vi "Autonomous.vi"   [LabVIEW 2018]
doc: "This VI starts when autonomous period begins, and will automatically be terminated when it ends. You can carry out timed or sensor driven operations directly to I/O or to subsystems without needing to return to the caller."
uses:
  <vilib>/Rock Robotics/WPI/Solenoid/WPI_SolenoidValue.ctl
  <vilib>/Rock Robotics/WPI/Utilities/WPI_GetSetVariantRefNum.vi
  <vilib>/Rock Robotics/Network Tables/NT Read String.vi
  Framework/Robot Global Data.vi
types:
  T1 = typedef "WPI_JoystickDevRef.ctl" = cluster{"Device":T2}
  T2 = typedef "WPI_JoystickDeviceEnum.ctl" = enum16{"USB 0", "USB 1", "USB 2", "USB 3", "USB 4", "USB 5"}
  T3 = typedef "WPI_SolenoidValue.ctl" = enum16{"Off", "On", "Forward", "Reverse"}
  T4 = typedef "Command Status Info.ctl" = cluster{"Name":string, "Status":T5, "notifier out":T6}
  T5 = typedef "Completion Status.ctl" = enum16{"Successful", "Aborted", "Incomplete"}
  T6 = typedef "Completion Notifier.ctl" = refnum<notifier>
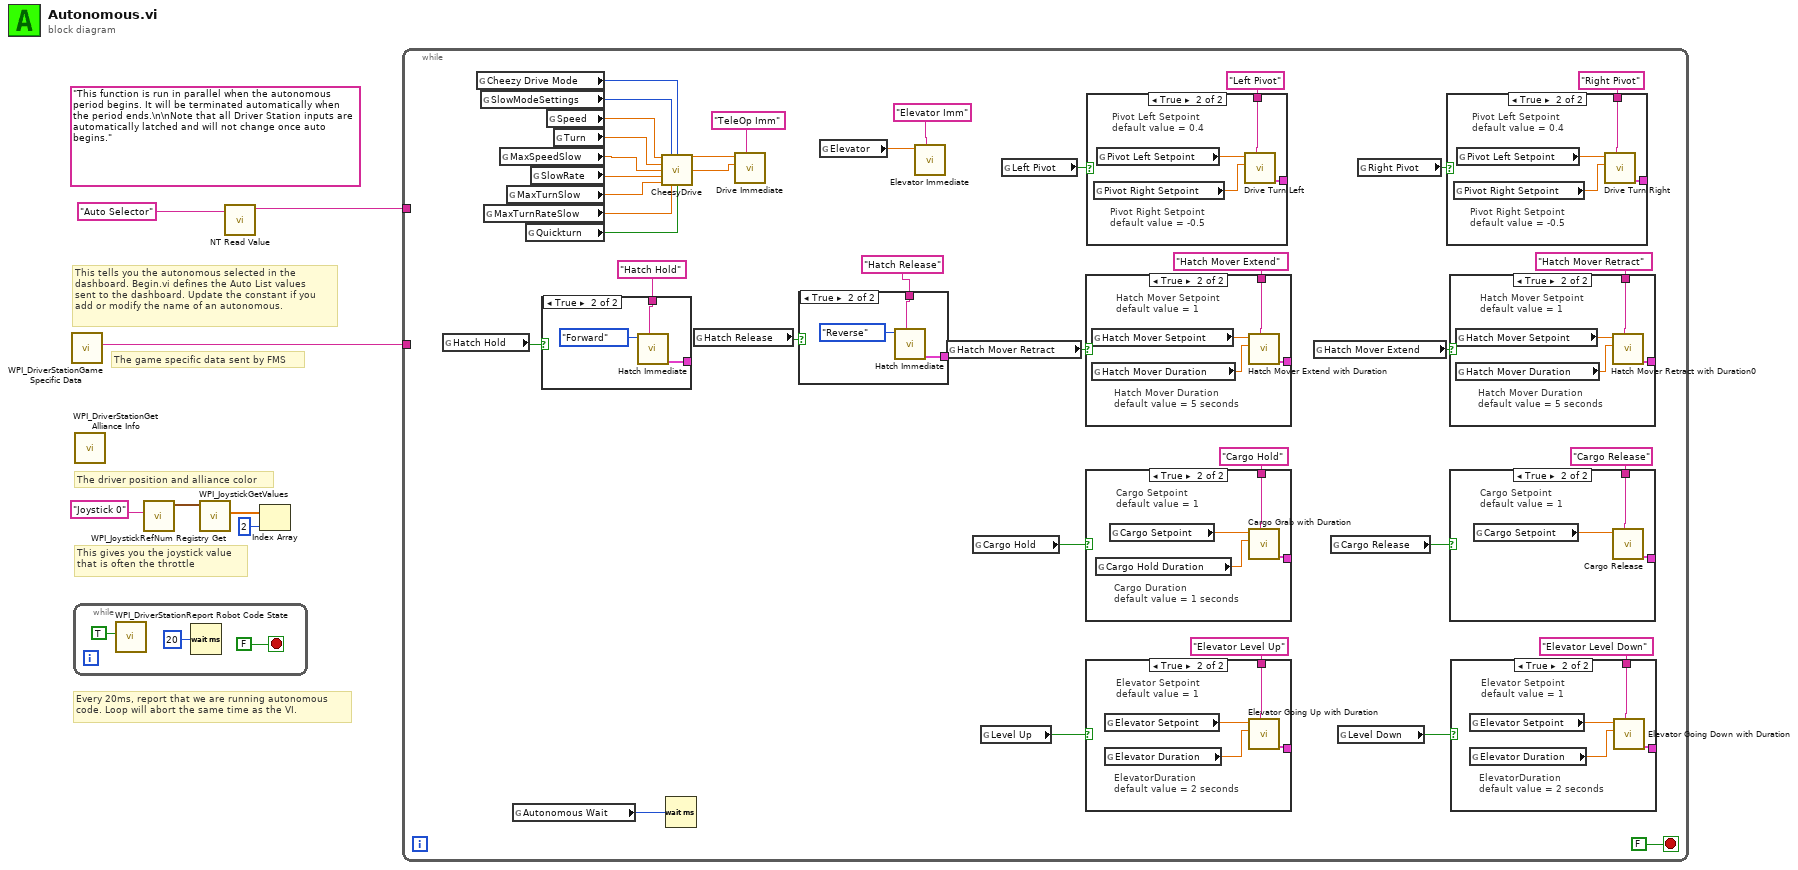
[diagram p0: block diagram]
diagram:
  (unwired) "This function is run in parallel when the autonomous period begins. It will be terminated automatically when the period ends.\n\nNote that all Driver Station inputs are automatically latched and will not change once auto begins."
  # "The game specific data sent by FMS"
  # "This tells you the autonomous selected in the \ndashboard. Begin.vi defines the Auto List values\nsent to the dashboard. Update the constant if you\nadd or modify the name of an autonomous."
  # "Every 20ms, report that we are running autonomous\ncode. Loop will abort the same time as the VI."
  # "This gives you the joystick value\nthat is often the throttle"
  # "The driver position and alliance color"
  n1 = call <vilib>:"WPI_DriverStationGame Specific Data.vi"() -> ("Game Specific Data"=w1:string)  [unwired: 11 in]
  n2 = while {
    stop <- FALSE stop-if-true
    n3 = call <vilib>:"WPI_DriverStationReport Robot Code State.vi"("Autonomous"=TRUE) -> ()  [unwired: 10 in, 1 out]
    n4 = Wait (ms)(milliseconds to wait=u32 20) -> ()  [unwired: 1 out]
  }
  n5 = call <vilib>:"WPI_DriverStationGet Alliance Info.vi"() -> ()  [unwired: 12 out]
  n6 = call <vilib>:"WPI_JoystickRefNum Registry Get.vi"("refnum name"="Joystick 0") -> ("JoystickDevRef"=w6:T1)  [unwired: 1 in, 9 out]
  n7 = call <vilib>:"WPI_JoystickGetValues.vi"("JoystickDevRef"=w6) -> ("Axes"=w5:dbl[])  [unwired: 6 in, 4 out]
  n8 = call-poly <vilib>:"NT Read Value.vi"("Name"="Auto Selector") -> ("String"=w2:string)  [unwired: 9 in, 1 out]
  n9 = Index Array(array=w5, index=2) -> ()  [unwired: 1 out]
  n10 = while {
    tunnel: w2 -> [_]
    tunnel: w1 -> [_]
    stop <- FALSE stop-if-true
    n11 = global read "Robot Global Data.vi" "Hatch Hold"() -> (w15:bool)
    n12 = global read "Robot Global Data.vi" "Cheezy Drive Mode"() -> (w34:u32)
    n13 = global read "Robot Global Data.vi" "SlowModeSettings"() -> (w35:i32)
    n14 = global read "Robot Global Data.vi" "MaxTurnRateSlow"() -> (w41:dbl)
    n15 = global read "Robot Global Data.vi" "MaxSpeedSlow"() -> (w38:dbl)
    n16 = global read "Robot Global Data.vi" "MaxTurnSlow"() -> (w40:dbl)
    n17 = global read "Robot Global Data.vi" "Autonomous Wait"() -> (w11:u32)
    n18 = global read "Robot Global Data.vi" "Quickturn"() -> (w42:bool)
    n19 = global read "Robot Global Data.vi" "SlowRate"() -> (w39:dbl)
    n20 = case shown="True" w15 {
      tunnel: [_ w82] -> _
      tunnel: "Hatch Hold" ("Description") -> [_ w81]
      frame False {
      }
      frame True {
        n21 = call "Hatch Immediate.vi"("Description"=w81, "Action"=WPI_SolenoidValue."Forward") -> ("Command Info Out"=w82:T4)  [unwired: 9 in]
      }
    }
    n22 = global read "Robot Global Data.vi" "Speed"() -> (w36:dbl)
    n23 = global read "Robot Global Data.vi" "Turn"() -> (w37:dbl)
    n24 = call "CheesyDrive.vi"("Throttle"=w36, "SlowModeSettings"=w35, "SlowMode"=w34, "Wheel"=w37, "MaxSpeedSlow"=w38, "SlowRate"=w39, "MaxTurnSlow"=w40, "MaxTurnRateSlow"=w41, "Quickturn"=w42) -> ("Left PWM"=w43:dbl, "Right PWM"=w44:dbl)  [unwired: 5 in]
    n25 = Wait (ms)(milliseconds to wait=w11) -> ()  [unwired: 1 out]
    n26 = global read "Robot Global Data.vi" "Hatch Release"() -> (w16:bool)
    n27 = call "Drive Immediate.vi"("Description"="TeleOp Imm", "Right Setpoint"=w44, "Left Setpoint"=w43) -> ()  [unwired: 8 in, 1 out]
    n28 = case shown="True" w16 {
      tunnel: [_ w79] -> _
      tunnel: "Hatch Release" ("Description") -> [_ w78]
      frame False {
      }
      frame True {
        n29 = call "Hatch Immediate.vi"("Description"=w78, "Action"=WPI_SolenoidValue."Reverse") -> ("Command Info Out"=w79:T4)  [unwired: 9 in]
      }
    }
    n30 = global read "Robot Global Data.vi" "Elevator"() -> (w46:dbl)
    n31 = call "Elevator Immediate.vi"("Description"="Elevator Imm", "Setpoint"=w46) -> ()  [unwired: 9 in, 1 out]
    n32 = global read "Robot Global Data.vi" "Hatch Mover Retract"() -> (w22:bool)
    n33 = global read "Robot Global Data.vi" "Cargo Hold"() -> (w27:bool)
    n34 = global read "Robot Global Data.vi" "Level Up"() -> (w30:bool)
    n35 = global read "Robot Global Data.vi" "Left Pivot"() -> (w19:bool)
    n36 = case shown="True" w22 {
      tunnel: "Hatch Mover Extend" ("Description") -> [_ w69]
      tunnel: [_ w66] -> _
      frame False {
      }
      frame True {
        # "Hatch Mover Duration\ndefault value = 5 seconds"
        # "Hatch Mover Setpoint\ndefault value = 1"
        n37 = global read "Robot Global Data.vi" "Hatch Mover Setpoint"() -> (w68:dbl)
        n38 = global read "Robot Global Data.vi" "Hatch Mover Duration"() -> (w67:dbl)
        n39 = call "Hatch Mover Extend with Duration.vi"("Description"=w69, "Duration (s)"=w67, "Setpoint"=w68) -> ("Command Info Out"=w66:T4)  [unwired: 8 in]
      }
    }
    n40 = case shown="True" w27 {
      tunnel: "Cargo Hold" ("Description") -> [_ w61]
      tunnel: [_ w58] -> _
      frame False {
      }
      frame True {
        # "Cargo Duration\ndefault value = 1 seconds"
        # "Cargo Setpoint\ndefault value = 1"
        n41 = global read "Robot Global Data.vi" "Cargo Hold Duration"() -> (w59:dbl)
        n42 = global read "Robot Global Data.vi" "Cargo Setpoint"() -> (w60:dbl)
        n43 = call "Cargo Grab with Duration.vi"("Description"=w61, "Duration (s)"=w59, "Setpoint"=w60) -> ("Command Info Out"=w58:T4)  [unwired: 8 in]
      }
    }
    n44 = case shown="True" w30 {
      tunnel: "Elevator Level Up" ("Description") -> [_ w54]
      tunnel: [_ w51] -> _
      frame False {
      }
      frame True {
        # "ElevatorDuration\ndefault value = 2 seconds"
        # "Elevator Setpoint\ndefault value = 1"
        n45 = global read "Robot Global Data.vi" "Elevator Setpoint"() -> (w53:dbl)
        n46 = global read "Robot Global Data.vi" "Elevator Duration"() -> (w52:dbl)
        n47 = call "Elevator Going Up with Duration.vi"("Description"=w54, "Duration (s)"=w52, "Setpoint"=w53) -> ("Command Info Out"=w51:T4)  [unwired: 8 in]
      }
    }
    n48 = case shown="True" w19 {
      tunnel: "Left Pivot" ("Description") -> [_ w77]
      tunnel: [_ w74] -> _
      frame False {
      }
      frame True {
        # "Pivot Right Setpoint\ndefault value = -0.5"
        # "Pivot Left Setpoint\ndefault value = 0.4"
        n49 = global read "Robot Global Data.vi" "Pivot Right Setpoint"() -> (w75:dbl)
        n50 = global read "Robot Global Data.vi" "Pivot Left Setpoint"() -> (w76:dbl)
        n51 = call "Drive Turn Left.vi"("Description"=w77, "Right Setpoint"=w75, "Left Setpoint"=w76) -> ("Command Info Out"=w74:T4)  [unwired: 8 in]
      }
    }
    n52 = global read "Robot Global Data.vi" "Hatch Mover Extend"() -> (w25:bool)
    n53 = global read "Robot Global Data.vi" "Cargo Release"() -> (w28:bool)
    n54 = global read "Robot Global Data.vi" "Level Down"() -> (w33:bool)
    n55 = global read "Robot Global Data.vi" "Right Pivot"() -> (w20:bool)
    n56 = case shown="True" w20 {
      tunnel: "Right Pivot" ("Description") -> [_ w73]
      tunnel: [_ w70] -> _
      frame False {
      }
      frame True {
        # "Pivot Right Setpoint\ndefault value = -0.5"
        # "Pivot Left Setpoint\ndefault value = 0.4"
        n57 = global read "Robot Global Data.vi" "Pivot Right Setpoint"() -> (w71:dbl)
        n58 = global read "Robot Global Data.vi" "Pivot Left Setpoint"() -> (w72:dbl)
        n59 = call "Drive Turn Right.vi"("Description"=w73, "Right Setpoint"=w71, "Left Setpoint"=w72) -> ("Command Info Out"=w70:T4)  [unwired: 8 in]
      }
    }
    n60 = case shown="True" w25 {
      tunnel: "Hatch Mover Retract" ("Description") -> [_ w65]
      tunnel: [_ w62] -> _
      frame False {
      }
      frame True {
        # "Hatch Mover Duration\ndefault value = 5 seconds"
        # "Hatch Mover Setpoint\ndefault value = 1"
        n61 = global read "Robot Global Data.vi" "Hatch Mover Setpoint"() -> (w64:dbl)
        n62 = global read "Robot Global Data.vi" "Hatch Mover Duration"() -> (w63:dbl)
        n63 = call "Hatch Mover Retract with Duration0.vi"("Description"=w65, "Duration (s)"=w63, "Setpoint"=w64) -> ("Command Info Out"=w62:T4)  [unwired: 8 in]
      }
    }
    n64 = case shown="True" w28 {
      tunnel: "Cargo Release" ("Description") -> [_ w57]
      tunnel: [_ w55] -> _
      frame False {
      }
      frame True {
        # "Cargo Setpoint\ndefault value = 1"
        n65 = global read "Robot Global Data.vi" "Cargo Setpoint"() -> (w56:dbl)
        n66 = call "Cargo Release.vi"("Description"=w57, "Setpoint"=w56) -> ("Command Info Out"=w55:T4)  [unwired: 9 in]
      }
    }
    n67 = case shown="True" w33 {
      tunnel: "Elevator Level Down" ("Description") -> [_ w50]
      tunnel: [_ w47] -> _
      frame False {
      }
      frame True {
        # "ElevatorDuration\ndefault value = 2 seconds"
        # "Elevator Setpoint\ndefault value = 1"
        n68 = global read "Robot Global Data.vi" "Elevator Setpoint"() -> (w49:dbl)
        n69 = global read "Robot Global Data.vi" "Elevator Duration"() -> (w48:dbl)
        n70 = call "Elevator Going Down with Duration.vi"("Description"=w50, "Duration (s)"=w48, "Setpoint"=w49) -> ("Command Info Out"=w47:T4)  [unwired: 8 in]
      }
    }
  }
